vi "RT Driver VI.vi"(6 "Device Clock":string, 9 "Device Inputs FIFO":refnum<k33>, 10 "Device Outputs FIFO":refnum<k33>, 11 "Device Reference":T1 format="%.0x") -> ()   [LabVIEW 2016, in "UDP Custom Device Engine.lvlib"]
uses:
  UDP Custom Device Engine.lvlib
  <vilib>/NI Veristand/Custom Device API/Custom Device Item Ref.ctl
  <vilib>/NI Veristand/Custom Device API/Custom Device Channel Type.ctl
  <vilib>/NI Veristand/Custom Device API/Get Item Property (U16).vi
  <vilib>/NI Veristand/Custom Device API/Get Item Property (String).vi
  Shared/Constants.vi
  <vilib>/NI Veristand/Custom Device API/Custom Device API.lvlib
  <vilib>/NI Veristand/Custom Device Tools/Custom Device Utility Library/Custom Device Utility Library.lvlib
  Shared/UDP Custom Device Shared.lvlib
panel:
  in  "Initialization Status Notifier":refnum<notifier>
  in  "Status Notifier":refnum<notifier>
  # "Custom Device Template\nv1.0"
  # "Use this template as a starting point for creating a custom device code module. The input controls shown here are specially named controls that the system will use to provide the device loop with data. The controls are not required for the device loop to run. For instance, if the device doesn't produce any output data, then you don't need the Device Outputs FIFO control. If you do use these controls, however, they need to have these exact names to be functional."
  # "The optional status notifier element is used to notify the RT engine of the last state of the custom device, and to indicate the device has completed execution. If this control is not used, a default No Error value is returned to the system when the device finishes execution.\n\nNote: This error state is not checked until the system shuts down. Use an output status channel to send more immediate status values to the system."
  # "This optional input can be used to send the VeriStand Engine the final status of the custom device initalization process. If this control exists on the custom device front panel, the VeriStand Engine will wait for a status update before starting up. If the custom device reports an error, that will abort the execution of the current configuration in the VeriStand Engine.\n\nThis control can be deleted if the custom device does not need to send the initialization status update."
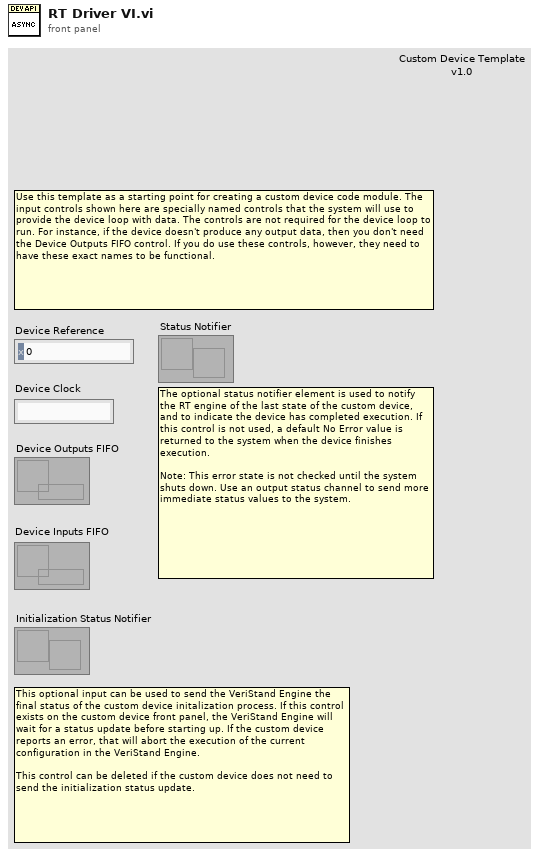
[diagram p1: front panel]
types:
  T1 = typedef "Custom Device API.lvlib/Custom Device Item Ref.ctl" = u64
  T2 = typedef "Custom Device API.lvlib/Custom Device Channel Type.ctl" = enum16{"Input", "Output"}
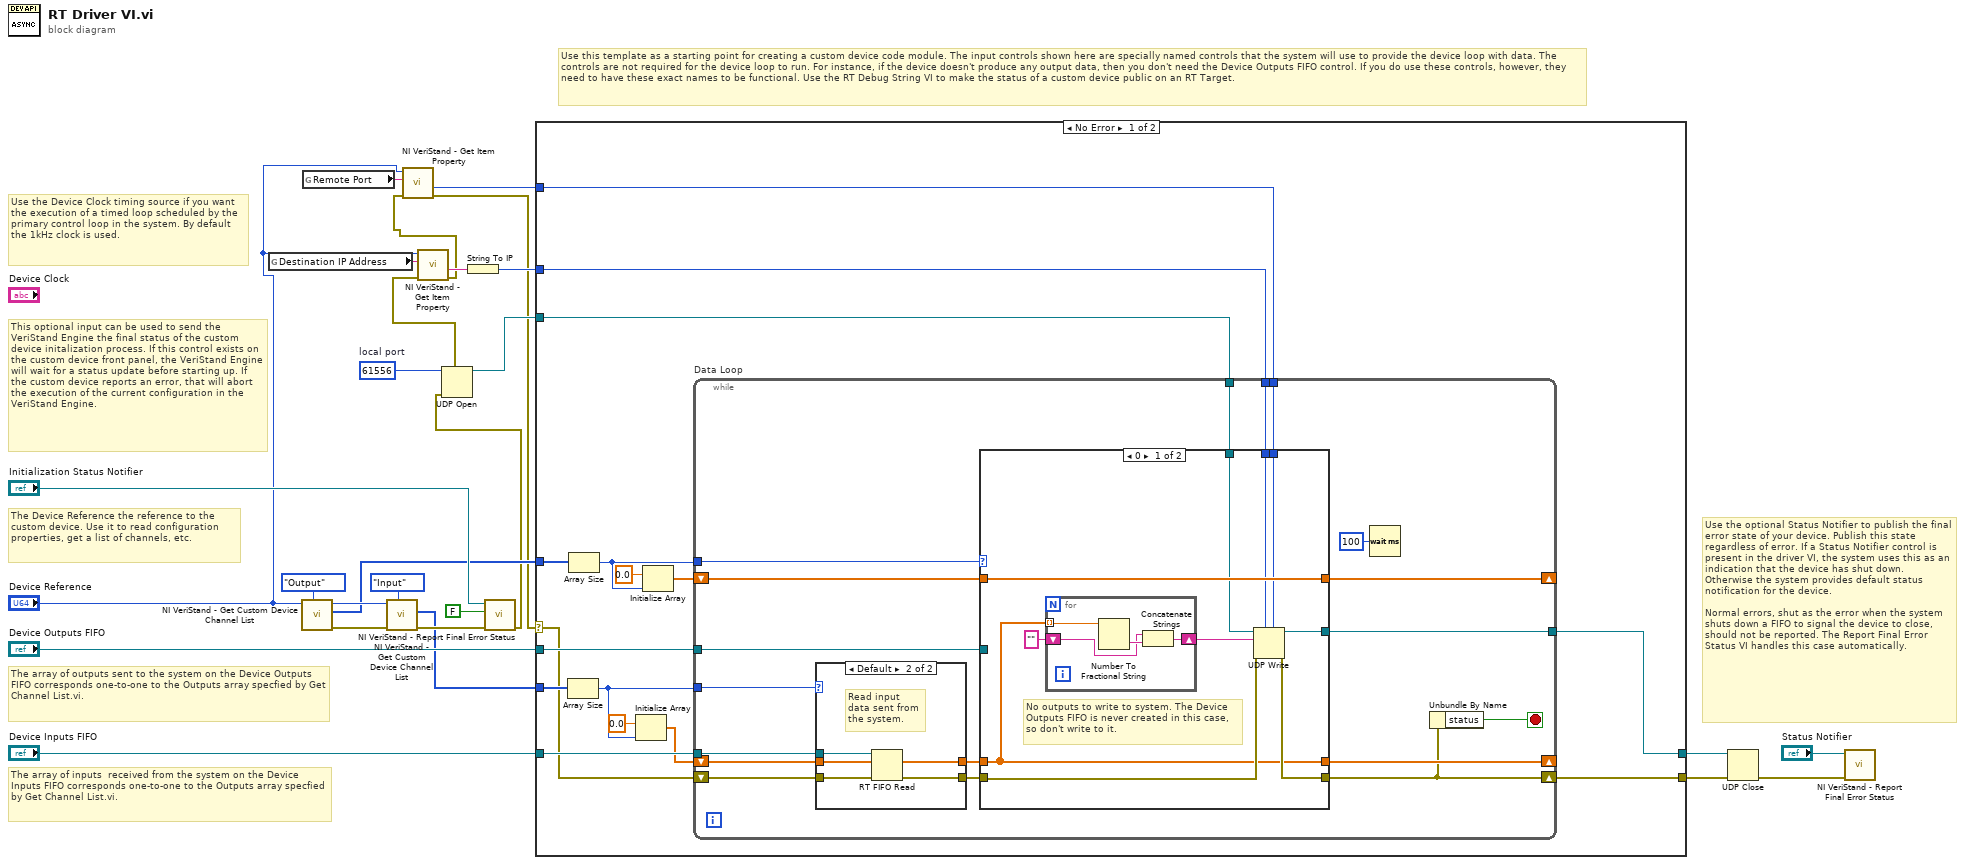
[diagram p0: block diagram]
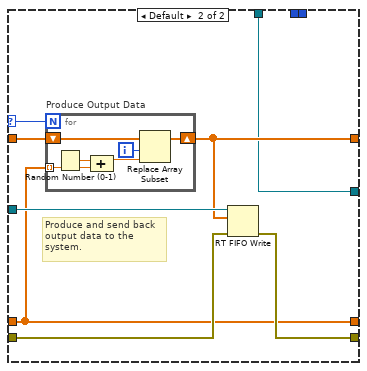
[diagram p2: hidden frame]
diagram:
  w13 = u16 61556  # local port
  # "This optional input can be used to send the VeriStand Engine the final status of the custom device initalization process. If this control exists on the custom device front panel, the VeriStand Engine will wait for a status update before starting up. If the custom device reports an error, that will abort the execution of the current configuration in the VeriStand Engine."
  # "The array of inputs  received from the system on the Device Inputs FIFO corresponds one-to-one to the Outputs array specfied by Get Channel List.vi."
  # "Use the optional Status Notifier to publish the final error state of your device. Publish this state regardless of error. If a Status Notifier control is present in the driver VI, the system uses this as an indication that the device has shut down. Otherwise the system provides default status notification for the device.\n\nNormal errors, shut as the error when the system shuts down a FIFO to signal the device to close, should not be reported. The Report Final Error Status VI handles this case automatically."
  # "The array of outputs sent to the system on the Device Outputs FIFO corresponds one-to-one to the Outputs array specfied by Get Channel List.vi."
  # "The Device Reference the reference to the custom device. Use it to read configuration properties, get a list of channels, etc."
  # "Use the Device Clock timing source if you want the execution of a timed loop scheduled by the primary control loop in the system. By default the 1kHz clock is used."
  # "Use this template as a starting point for creating a custom device code module. The input controls shown here are specially named controls that the system will use to provide the device loop with data. The controls are not required for the device loop to run. For instance, if the device doesn't produce any output data, then you don't need the Device Outputs FIFO control. If you do use these controls, however, they need to have these exact names to be functional. Use the RT Debug String VI to make the status of a custom device public on an RT Target."
  n1 = global read "Constants.vi" "Destination IP Address"() -> (w7:string)
  n2 = call <vilib>:"NI VeriStand - Get Custom Device Channel List.vi"("Channel Type"=Custom_Device_Channel_Type."Output", "Device Ref in"="Device Reference") -> ("error out"=w21:errorcluster, "Specified Channel Ref List"=w18:T1[], "Device Ref out"=w22:T1)  [unwired: 1 in, 6 out]
  n3 = global read "Constants.vi" "Remote Port"() -> (w8:string)
  n4 = call <vilib>:"NI VeriStand - Get Custom Device Channel List.vi"("Channel Type"=Custom_Device_Channel_Type."Input", "error in (no error)"=w21, "Device Ref in"=w22) -> ("error out"=w27:errorcluster, "Specified Channel Ref List"=w19:T1[])  [unwired: 7 out]
  n5 = call <vilib>:"NI VeriStand - Report Final Error Status.vi"("error in (no error)"=w27, "Filter FIFO & Shutdown Errors (T)"=FALSE ("Filter FIFO Errors (T)"), "Status Notifier"="Initialization Status Notifier") -> ("error out"=w10:errorcluster)  [unwired: 8 out]
  n6 = UDP Open(8:w10, 11:w13) -> (port=w11:refnum<k16>, 0:w3:errorcluster)  [unwired: 3 in, 1 out]
  n7 = call-poly <vilib>:"NI VeriStand - Get Item Property.vi"("error in (no error)"=w3, "Property Name"=w7, "Item Ref in"="Device Reference") -> ("error out"=w2:errorcluster, "Value"=w6:string)  [unwired: 5 in, 2 out]
  n8 = call-poly <vilib>:"NI VeriStand - Get Item Property.vi"("error in (no error)"=w2, "Property Name"=w8, "Item Ref in"="Device Reference") -> ("error out"=w1:errorcluster, "Value"=w5:u16)  [unwired: 5 in, 2 out]
  n9 = String To IP(1:w6) -> (0:w12:u32)
  n10 = case shown="No Error" w1 {
    selector: w1 -> [w33 w98]
    tunnel: "Device Outputs FIFO" -> [w43 _]
    tunnel: "Device Inputs FIFO" -> [w42 _]
    tunnel: w19 -> [w36 _]
    tunnel: w18 -> [w35 _]
    tunnel: [w32 w98] -> w15
    tunnel: w5 -> [w31 _]
    tunnel: w12 -> [w30 _]
    tunnel: w11 -> [w29 w97]
    tunnel: [w28 w97] -> w9
    frame No Error {
      n11 = Array Size(array=w36) -> (size(s)=w34:i32)
      n12 = Array Size(array=w35) -> (size(s)=w37:i32)
      n13 = Initialize Array(0.0 ("element"), w34) -> (w38:dbl[])
      n14 = Initialize Array(0.0 ("element"), w37) -> (w39:dbl[])
      n15 = while "Data Loop" {
        shift-right: [w59] -> _
        shift-left: w38 -> [w60]
        shift-right: [w52] -> w32
        shift-left: w33 -> [w61]
        shift-right: [w57] -> _
        shift-left: w39 -> [w58]
        tunnel: w37 -> [w54]
        tunnel: w43 -> [w56]
        tunnel: w42 -> [w55]
        tunnel: w34 -> [w53]
        tunnel: w31 -> [w51]
        tunnel: w30 -> [w50]
        tunnel: w29 -> [w49]
        tunnel: [w48] -> w28
        stop <- w44 stop-if-true
        n16 = case shown="Default" w53 {
          tunnel: w55 -> [_ w96]
          tunnel: w60 -> [w91 w95]
          tunnel: [w91 w94] -> w47
          tunnel: [w90 w93] -> w46
          tunnel: w61 -> [w90 w92]
          frame 0 {
            # "No inputs to read\nfrom system. Inputs FIFO not created in this case, so don't write to it."
          }
          frame Default {
            # "Read input data sent from the system."
            n17 = RT FIFO Read(0:w96, 1:w95, 3:w92) -> (9:w94:dbl[], 11:w93:errorcluster)  [unwired: 4 out]
          }
        }
        n18 = case shown="0" w54 {
          selector: w54 -> [_ w77]
          tunnel: w56 -> [_ w83]
          tunnel: w58 -> [w71 w82]
          tunnel: w47 -> [w66 w78]
          tunnel: w46 -> [w68 w81]
          tunnel: [w67 w80] -> w52
          tunnel: [w71 w79] -> w57
          tunnel: [w66 w78] -> w59
          tunnel: w51 -> [w65 _]
          tunnel: w50 -> [w64 _]
          tunnel: w49 -> [w63 w76]
          tunnel: [w62 w76] -> w48
          frame 0 {
            # "No outputs to write to system. The Device Outputs FIFO is never created in this case, so don't write to it."
            n19 = for {
              shift-right: [w74] -> w70
              shift-left: "" -> [w73]
              tunnel: w66 -> [w72] mode=indexing
              n20 = Number To Fractional String(number=w72) -> (F-format string=w75:string)  [unwired: 3 in]
              n21 = Concatenate Strings(w73, w75) -> (w74:string)
            }
            n22 = UDP Write(address=w64, port or service name=w65, connection ID=w63, data in=w70, 8:w68) -> (error out=w67:errorcluster, 3:w62:refnum<k16>)  [unwired: 1 in]
          }
          frame Default {
            # "Produce and send back output data to the system."
            n23 = for "Produce Output Data" {
              N: w77 -> [_]
              shift-right: [w88] -> w79
              shift-left: w82 -> [w89]
              tunnel: w78 -> [w84] mode=indexing
              i -> [w87]
              n24 = Random Number (0-1)() -> (number: 0 to 1=w86:dbl)
              n25 = Compound Arithmetic op=ADD(w86, w84) -> (w85:dbl)
              n26 = Replace Array Subset(array=w89, new element=w85, index=w87) -> (w88:dbl[])
            }
            n27 = RT FIFO Write(0:w83, 1:w79, 3:w81) -> (11:w80:errorcluster)  [unwired: 1 in, 4 out]
          }
        }
        n28 = Wait (ms)(milliseconds to wait=u32 100) -> ()  [unwired: 1 out]
        n29 = Unbundle By Name(w52) -> ("status"=w44:bool)
      }
    }
    frame Error {
    }
  }
  n30 = UDP Close(connection ID=w9, 8:w15) -> (error out=w14:errorcluster)  [unwired: 1 out]
  n31 = call <vilib>:"NI VeriStand - Report Final Error Status.vi"("error in (no error)"=w14, "Status Notifier"="Status Notifier") -> ()  [unwired: 1 in, 9 out]
